vi "parse_point_cloud2.vi"(4 "error in":errorcluster, 7 "msg in":string) -> (0 "error out":errorcluster, 1 "PointCloud2":T1, 2 "Header":T2, 3 "msg out":string)   [LabVIEW 2015]
uses:
  std_msgs/subs/parse_u32_scalar.vi
  std_msgs/subs/parse_bool_scalar.vi
  std_msgs/subs/parse_u8_scalar.vi
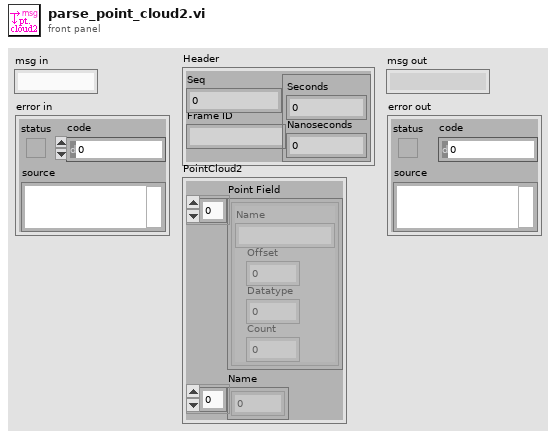
[diagram p1: front panel]
types:
  T1 = cluster{"Point Field":cluster{"Name":string, "Offset":u32, "Datatype":u8, "Count":u32}[], "Name":u8[]}
  T2 = cluster{"Seq":u32, "Frame ID":string, cluster{"Seconds":i32, "Nanoseconds":i32}}
  T3 = cluster{"Seq":u32, "Frame ID":string, "Timestamp":cluster{"Seconds":i32, "Nanoseconds":i32}}
  T4 = cluster{"Name":string, "Offset":u32, "Datatype":u8, "Count":u32}
  T5 = cluster{cluster{"Name":string, "Offset":u32, "Datatype":u8, "Count":u32}[], u8[]}
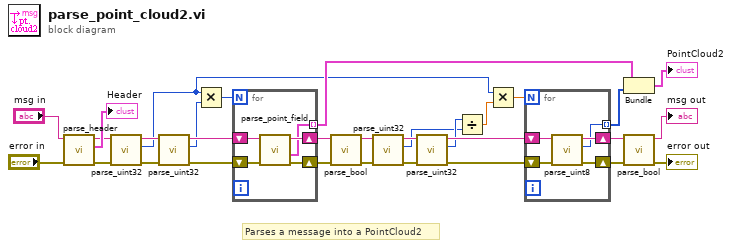
[diagram p0: block diagram]
diagram:
  # "Parses a message into a PointCloud2"
  n1 = call "parse_header.vi"("error in"="error in", "msg in"="msg in") -> ("error out"=w27:errorcluster, "Header"=→"Header":T3, "msg out"=w26:string)  [unwired: 3 in]
  n2 = call-poly "parse_uint32.vi"("error in"=w27, "msg in"=w26) -> ("error out"=w28:errorcluster, "number"=w2:u32, "msg out"=w25:string)  [unwired: 3 in]
  n3 = call-poly "parse_uint32.vi"("error in"=w28, "msg in"=w25) -> ("error out"=w16:errorcluster, "number"=w10:u32, "msg out"=w24:string)  [unwired: 3 in]
  n4 = Multiply(x=w2, y=w10) -> (x*y=w9:u32)
  n5 = for {
    N: w9 -> [_]
    shift-right: [w35] -> w23
    shift-left: w24 -> [w36]
    shift-right: [w33] -> w15
    shift-left: w16 -> [w34]
    tunnel: [w32] -> w8 mode=indexing
    n6 = call "parse_point_field.vi"("error in"=w34, "msg in"=w36) -> ("error out"=w33:errorcluster, "PointField"=w32:T4, "msg out"=w35:string)  [unwired: 2 in, 1 out]
  }
  n7 = call-poly "parse_bool.vi"("error in"=w15, "msg in"=w23) -> ("error out"=w14:errorcluster, "msg out"=w22:string)  [unwired: 3 in, 1 out]
  n8 = call-poly "parse_uint32.vi"("error in"=w14, "msg in"=w22) -> ("error out"=w13:errorcluster, "number"=w4:u32, "msg out"=w21:string)  [unwired: 3 in]
  n9 = call-poly "parse_uint32.vi"("error in"=w13, "msg in"=w21) -> ("error out"=w12:errorcluster, "number"=w5:u32, "msg out"=w20:string)  [unwired: 3 in]
  n10 = Divide(x=w5, y=w4) -> (x/y=w3:dbl)
  n11 = Multiply(x=w2, y=w3) -> (x*y=w1:dbl)
  n12 = for {
    N: w1 -> [_]
    shift-right: [w41] -> w19
    shift-left: w20 -> [w40]
    shift-right: [w38] -> w11
    shift-left: w12 -> [w39]
    tunnel: [w37] -> w7 mode=indexing
    n13 = call-poly "parse_uint8.vi"("error in"=w39, "msg in"=w40) -> ("error out"=w38:errorcluster, "number"=w37:u8, "msg out"=w41:string)  [unwired: 3 in]
  }
  n14 = Bundle(w8, w7) -> (→"PointCloud2":T5)  [unwired: 1 in]
  n15 = call-poly "parse_bool.vi"("error in"=w11, "msg in"=w19) -> ("error out"=→"error out":errorcluster, "msg out"=→"msg out":string)  [unwired: 3 in, 1 out]
